vi "Tests Launcher.vi"(8 "Error In":errorcluster) -> (0 "Error Out":errorcluster)   [LabVIEW 2015, in "unit tests.lvlib"]
uses:
  unit tests.lvlib
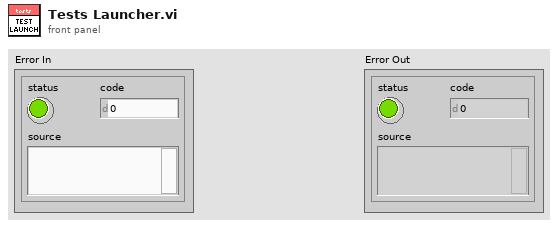
[diagram p1: front panel]
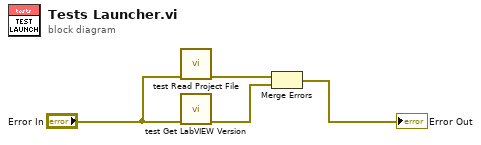
[diagram p0: block diagram]
diagram:
  n1 = call "test Read Project File.vi"("Error In"="Error In") -> ("Error Out"=w3:errorcluster)  [unwired: 10 in]
  n2 = call "test Get LabVIEW Version.vi"("Error In"="Error In") -> ("Error Out"=w2:errorcluster)  [unwired: 10 in]
  n3 = Merge Errors(w3, w2) -> (→"Error Out":errorcluster)
